vi "PTScanner.dialog edit object.vi"(0 "object ref":refnum<vi>, 2 "Parameters In":T1, 4 "new":bool) -> (14 "object ref out":refnum<vi>, 16 "Parameters Out":T1, 18 "changed":bool)   [LabVIEW 2014, in "PTScanner.lvlib"]
uses:
  PTScanner.lvlib
  _typedefs/scan method parameters/scan method parameters.xctl
  PTScanner.obj parameters.ctl
  _common/PTUtils/PTUtils.lvlib
panel:
  in  "Update button":bool
  in  "different channels":bool caption="diff Channels"
  in  "Channel":i32=-1
  in  "lock address":bool=TRUE caption="locked"
  in  "Range":dbl=1e-15
  in  "dataDescriptor":string caption="Act. Value Service Name"
  in  "cancel":bool
  in  "ok":bool
  in  "Call Mode":enum16{"Simple DIM", "Synchronous"}(ring) caption="Call"
  in  "DIM Services":u16(ring) caption="Services" items=["AG33250A_accessID", "AG33250A_actAmplitude", "AG33250A_actBurstEnabled", "AG33250A_actCycles", "AG33250A_actDCOffset", "AG33250A_actFrequency", "AG33250A_actOutputEnabled", "AG33250A_actPeriod", "AG33250A_actPhase", "AG33250A_actTrigger", "AG33250A_actTriggerDelay", "AG33250A_actWaveform", "AG33250A_birthday", "AG33250A_classID", "AG33250A_condition", "AG33250A_deviceGUI", "AG33250A_deviceID", "AG33250A_deviceState", "AG33250A_eventError", "AG33250A_eventStatus", "AG33250A_evtCounter", "AG33250A_nomAmplitude", "AG33250A_nomBurstEnabled", "AG33250A_nomCycles", "AG33250A_nomDCOffset", "AG33250A_nomFrequency", "AG33250A_nomOutputEnabled", "AG33250A_nomPeriod", "AG33250A_nomPhase", "AG33250A_nomTrigger", "AG33250A_nomTriggerDelay", "AG33250A_nomWaveform", "AG33250A_pdcCounter", "AG33250A_periodicError", "AG33250A_periodicStatus", "AG33250A_systemID", "AG33250A_watchdog"]
  in  "DIM Service":string caption="Act. Value Service Name"
  in  "Method":u16(ring) items=["Ping", "GetDescriptors", "SetPdcInterval", "SetPdcPreset", "SetEvtPreset", "GetEvtStatus", "GetCNames", "GetIList", "Reset", "ReadData", "STOP", "Wait", "WakeupPeriodic", "GetVersionOfLibrary", "Initialize", "Close", "IDQuery", "SetAdvancedGUI", "SetGauss", "UseAM", "ErrorQuery", "SetFrequency", "SetAmplitude", "SetDCOffset", "SetTrigger", "SetBurst", "SetOutputEnabled", "SendTrigger"]
  in  "Object":u16(ring) items=["AG33250A"]
  in  "Step":dbl=1e-15 min=1e-15
  in  "Plus":dbl
  in  "Minus":dbl
  in  "Centroid":dbl
  in  "Method Parameters":T2(xcontrol) caption="Method Input Parameters"
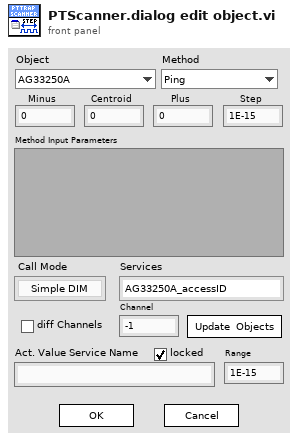
[diagram p1: front panel]
types:
  T1 = typedef "PTScanner.lvlib/PTScanner.obj parameters.ctl" = cluster{"object":string, "DIM address":string, "method":string, "data descriptor":string, "method parameters":cluster{"Name":string, "Descr":string, "Value":string, "Value?":bool}[], "Call Mode":enum16{"Simple DIM", "Synchronous"}, "actValue":dbl, "Centroid":dbl, "Minus Delta":dbl, "Plus Delta":dbl, "increment":dbl, "DIM Status":cluster{"no link":bool, "quality":i32, "Time Stamp":timestamp}, "range":dbl, "DIMChannelIndex":i32}
  T2 = cluster{"Name":string, "Descr":string, "Value":string, "Value?":bool}[]
  T3 = enum8{"Enabled", "Disabled", "Disabled and Grayed Out"}
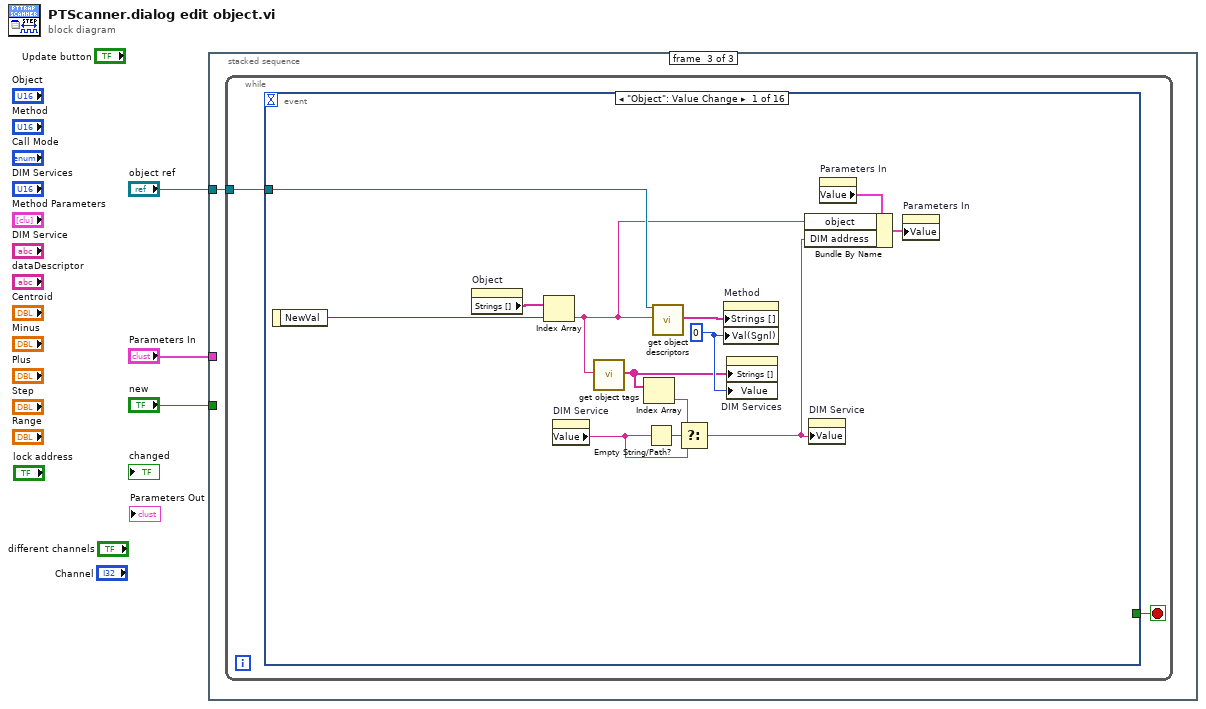
[diagram p0: block diagram]
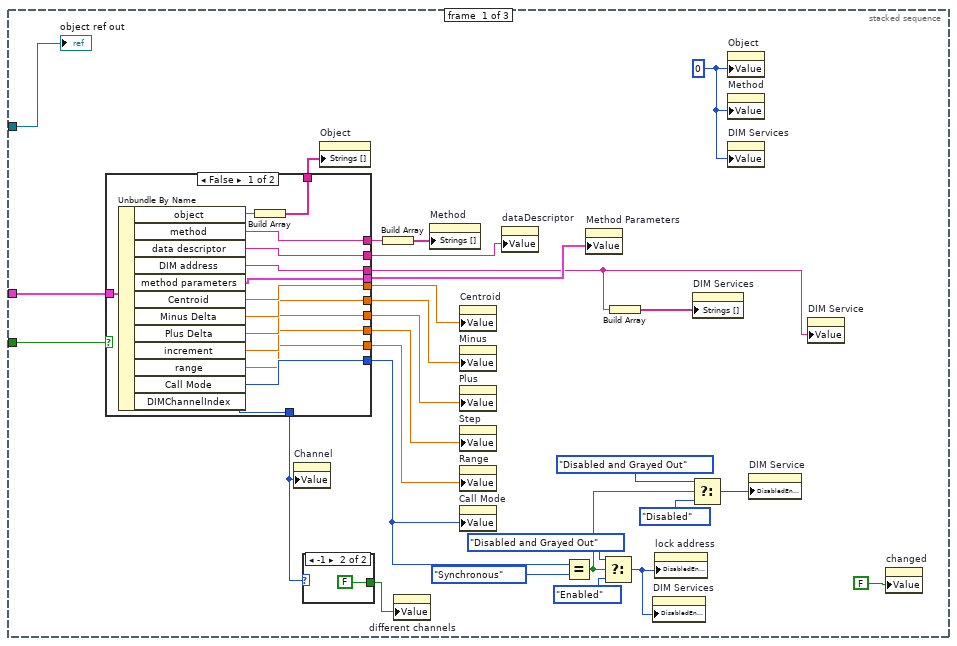
[diagram p2: hidden frame]
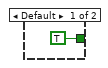
[diagram p3: hidden frame]
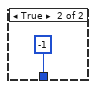
[diagram p4: hidden frame]
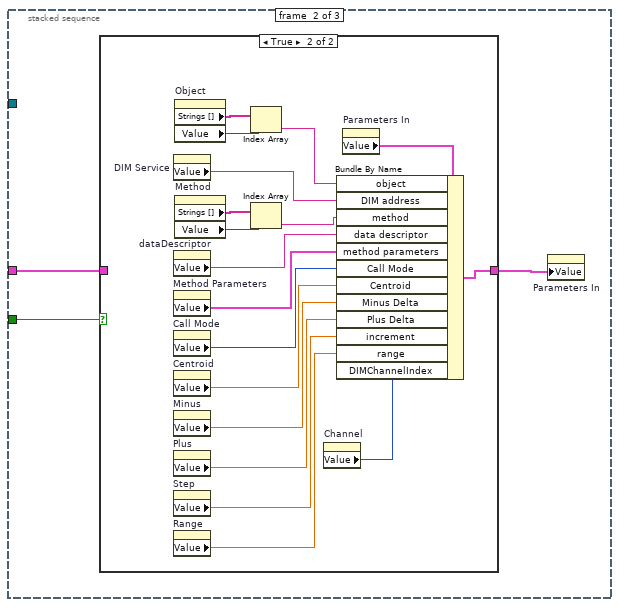
[diagram p5: hidden frame]
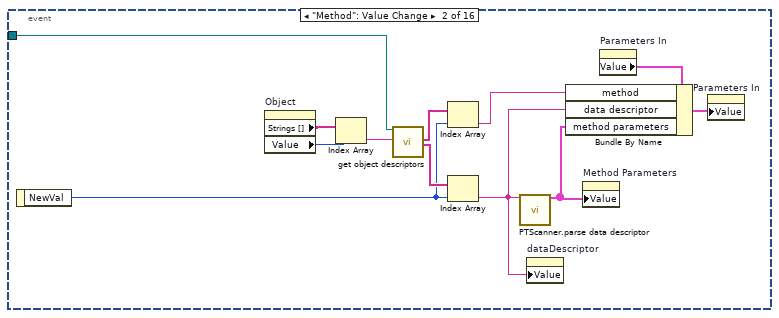
[diagram p7: hidden frame]
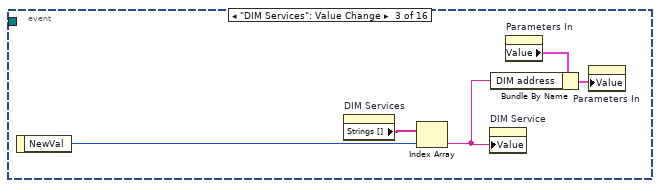
[diagram p8: hidden frame]
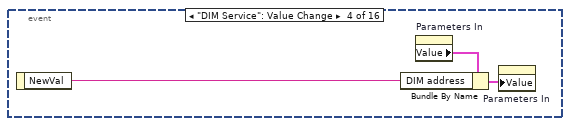
[diagram p9: hidden frame]
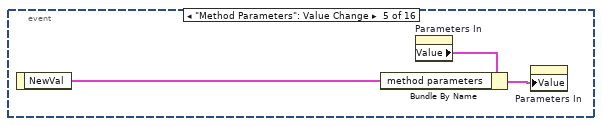
[diagram p10: hidden frame]
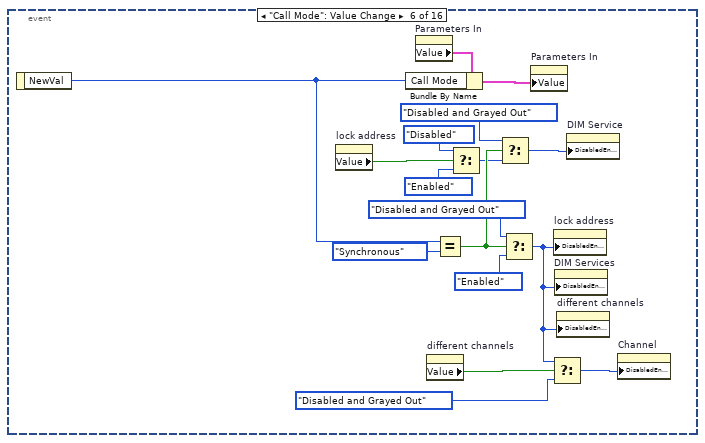
[diagram p11: hidden frame]
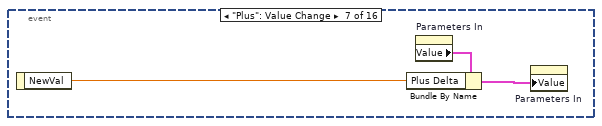
[diagram p12: hidden frame]
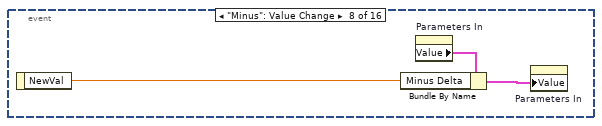
[diagram p13: hidden frame]
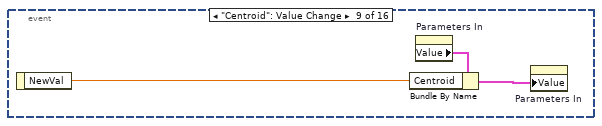
[diagram p14: hidden frame]
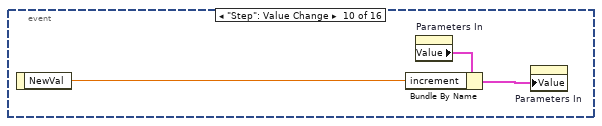
[diagram p15: hidden frame]
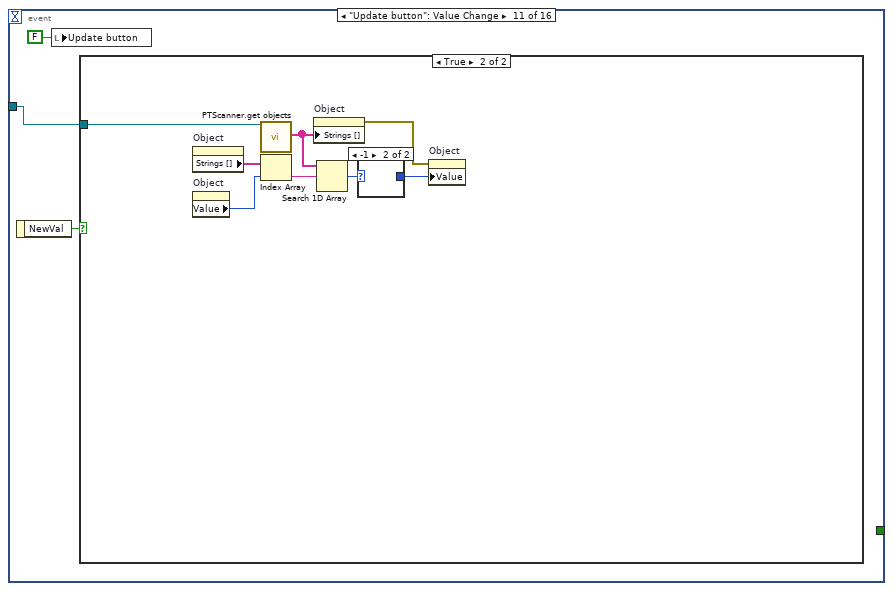
[diagram p16: hidden frame]
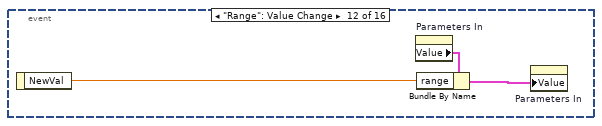
[diagram p19: hidden frame]
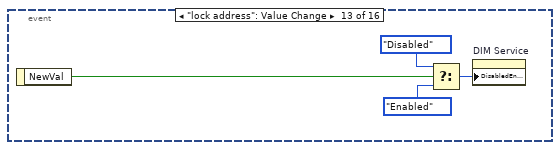
[diagram p20: hidden frame]
diagram:
  n1 = stacked-sequence {
    tunnel: "new" -> [w14 w51 _]
    tunnel: "object ref" -> [w25 _ w71]
    tunnel: "Parameters In" -> [w31 w50 _]
    frame #0 {
      w6 = 0
      n2 = case shown="False" w14 {
        tunnel: w31 -> [w40 _]
        tunnel: [w47 _] -> w10
        tunnel: [w46 _] -> w8
        tunnel: [w45 _] -> w4
        tunnel: [w44 _] -> w30
        tunnel: [w43 _] -> w27
        tunnel: [w42 _] -> w28
        tunnel: [w41 _] -> w29
        tunnel: [w39 _] -> w21
        tunnel: [w38 _] -> w20
        tunnel: [w37 _] -> w7
        tunnel: [w36 -1 ("DIMChannelIndex")] -> w13
        tunnel: [w34 _] -> w11
        frame False {
          n3 = Unbundle By Name(w40) -> ("object"=w35:string, "method"=w47:string, "data descriptor"=w46:string, "DIM address"=w45:string, "method parameters"=w37:T2, "Centroid"=w44:dbl, "Minus Delta"=w43:dbl, "Plus Delta"=w42:dbl, "increment"=w41:dbl, "range"=w38:dbl, "Call Mode"=w39:enum16{"Simple DIM", "Synchronous"}, "DIMChannelIndex"=w36:i32)
          n4 = Build Array(w35) -> (w34:string[])
        }
        frame True {
        }
      }
      n5 = property on="Channel" class="DigNum (strict)"("Value"=w13) -> ()  [unwired: 2 in, 2 out]
      n6 = case shown="-1" w13 {
        tunnel: [TRUE ("changed") FALSE ("changed")] -> w12
        frame Default {
        }
        frame -1 {
        }
      }
      n7 = property on="Object" class="Ring (strict)"("Strings []"=w11) -> ()  [unwired: 2 in, 2 out]
      n8 = Build Array(w10) -> (w9:string[])
      n9 = property on="different channels" class="Bool (strict)"("Value"=w12) -> ()  [unwired: 2 in, 2 out]
      n10 = property on="Method" class="Ring (strict)"("Strings []"=w9) -> ()  [unwired: 2 in, 2 out]
      n11 = property on="Centroid" class="DigNum (strict)"("Value"=w30) -> ()  [unwired: 2 in, 2 out]
      n12 = property on="Minus" class="DigNum (strict)"("Value"=w27) -> ()  [unwired: 2 in, 2 out]
      n13 = property on="Plus" class="DigNum (strict)"("Value"=w28) -> ()  [unwired: 2 in, 2 out]
      n14 = property on="Step" class="DigNum (strict)"("Value"=w29) -> ()  [unwired: 2 in, 2 out]
      n15 = property on="Range" class="DigNum (strict)"("Value"=w20) -> ()  [unwired: 2 in, 2 out]
      n16 = property on="Call Mode" class="Enum (strict)"("Value"=w21) -> ()  [unwired: 2 in, 2 out]
      n17 = property on="dataDescriptor" class="Str"("Value"=w8) -> ()  [unwired: 2 in, 2 out]
      n18 = Equal?(x=w21, y=enum16{"Simple DIM", "Synchronous"}."Synchronous" ("Call Mode")) -> (x = y?=w18:bool)
      n19 = property on="Method Parameters" class="scan method parameters (strict)"("Value"=w7) -> ()  [unwired: 2 in, 2 out]
      n20 = Select(t=T3."Disabled and Grayed Out" ("Disabled"), s=w18, f=T3."Enabled" ("Disabled")) -> (s? t:f=w19:T3)
      n21 = Build Array(w4) -> (w5:string[])
      n22 = property on="DIM Services" class="Ring (strict)"("DisabledEnum"=w19) -> ()  [unwired: 2 in, 2 out]
      n23 = property on="lock address" class="Bool (strict)"("DisabledEnum"=w19) -> ()  [unwired: 2 in, 2 out]
      n24 = Select(t=T3."Disabled and Grayed Out" ("Disabled"), s=w18, f=T3."Disabled" ("Disabled")) -> (s? t:f=w15:T3)
      n25 = property on="DIM Services" class="Ring (strict)"("Strings []"=w5) -> ()  [unwired: 2 in, 2 out]
      n26 = property on="Object" class="Ring (strict)"("Value"=w6) -> ()  [unwired: 2 in, 2 out]
      n27 = property on="Method" class="Ring (strict)"("Value"=w6) -> ()  [unwired: 2 in, 2 out]
      n28 = property on="DIM Services" class="Ring (strict)"("Value"=w6) -> ()  [unwired: 2 in, 2 out]
      n29 = property on="DIM Service" class="Str"("DisabledEnum"=w15) -> ()  [unwired: 2 in, 2 out]
      n30 = property on="DIM Service" class="Str"("Value"=w4) -> ()  [unwired: 2 in, 2 out]
      n31 = property on="changed" class="Bool (strict)"("Value"=FALSE ("changed")) -> ()  [unwired: 2 in, 2 out]
      "object ref out" <- w25
    }
    frame #1 {
      n32 = case shown="True" w51 {
        tunnel: w50 -> [w52 _]
        tunnel: [w52 w65] -> w49
        frame False {
        }
        frame True {
          n33 = property on="DIM Service" class="Str"() -> ("Value"=w63:string)  [unwired: 2 in, 2 out]
          n34 = property on="dataDescriptor" class="Str"() -> ("Value"=w61:string)  [unwired: 2 in, 2 out]
          n35 = property on="Method Parameters" class="scan method parameters (strict)"() -> ("Value"=w60:T2)  [unwired: 2 in, 2 out]
          n36 = property on="Call Mode" class="Enum (strict)"() -> ("Value"=w59:enum16{"Simple DIM", "Synchronous"})  [unwired: 2 in, 2 out]
          n37 = property on="Centroid" class="DigNum (strict)"() -> ("Value"=w58:dbl)  [unwired: 2 in, 2 out]
          n38 = property on="Minus" class="DigNum (strict)"() -> ("Value"=w57:dbl)  [unwired: 2 in, 2 out]
          n39 = property on="Plus" class="DigNum (strict)"() -> ("Value"=w56:dbl)  [unwired: 2 in, 2 out]
          n40 = property on="Step" class="DigNum (strict)"() -> ("Value"=w55:dbl)  [unwired: 2 in, 2 out]
          n41 = property on="Range" class="DigNum (strict)"() -> ("Value"=w54:dbl)  [unwired: 2 in, 2 out]
          n42 = property on="Object" class="Ring (strict)"() -> ("Strings []"=w70:string[], "Value"=w69:u16)  [unwired: 2 in, 2 out]
          n43 = property on="Method" class="Ring (strict)"() -> ("Strings []"=w68:string[], "Value"=w67:u16)  [unwired: 2 in, 2 out]
          n44 = Index Array(array=w70, index=w69) -> (element=w64:string)
          n45 = Index Array(array=w68, index=w67) -> (element=w62:string)
          n46 = property on="Channel" class="DigNum (strict)"() -> ("Value"=w53:i32)  [unwired: 2 in, 2 out]
          n47 = property on="Parameters In" class="Clust (strict)"() -> ("Value"=w66:T1)  [unwired: 2 in, 2 out]
          n48 = Bundle By Name(cluster=w66, "object"=w64, "DIM address"=w63, "method"=w62, "data descriptor"=w61, "method parameters"=w60, "Call Mode"=w59, "Centroid"=w58, "Minus Delta"=w57, "Plus Delta"=w56, "increment"=w55, "range"=w54, "DIMChannelIndex"=w53) -> (w65:T1)
        }
      }
      n49 = property on="Parameters In" class="Clust (strict)"("Value"=w49) -> ()  [unwired: 2 in, 2 out]
    }
    frame #2 {
      n50 = while {
        tunnel: w71 -> [w72]
        stop <- w73 stop-if-true
        n51 = event shown="[0] \"Object\": Value Change" {
          selector: _ -> [_ _ _ _ _ _ _ _ _ _ _ _ _ _ _ _]
          dyn-events: _ -> [_ _ _ _ _ _ _ _ _ _ _ _ _ _ _ _]
          timeout: _ -> [_ _ _ _ _ _ _ _ _ _ _ _ _ _ _ _]
          tunnel: [_ _ _ _ _ _ _ _ _ _ _ _ _ w158 "ok" "cancel"] -> w73
          tunnel: w72 -> [w79 w94 _ _ _ _ _ _ _ _ w139 _ _ _ _ _]
          event "Object": Value Change {
            w81 = u16 0
            n52 = event-data() -> ("NewVal"=w78:u16)  [unwired: 1 in]
            n53 = property on="Object" class="Ring (strict)"() -> ("Strings []"=w83:string[])  [unwired: 2 in, 2 out]
            n54 = Index Array(array=w83, index=w78) -> (element=w75:string)
            n55 = property on="DIM Service" class="Str"() -> ("Value"=w84:string)  [unwired: 2 in, 2 out]
            n56 = call "get object tags.vi"("Object"=w75) -> ("services"=w80:string[])  [unwired: 16 in, 2 out]
            n57 = Index Array(array=w80) -> (element=w85:string)  [unwired: 1 in]
            n58 = Empty String/Path?(string/path=w84) -> (empty?=w86:bool)
            n59 = call "get object descriptors.vi"("i ref in"=w79, "Object"=w75) -> ("selectors"=w82:string[])  [unwired: 14 in, 3 out]
            n60 = Select(t=w85, s=w86, f=w84) -> (s? t:f=w74:string)
            n61 = property on="Method" class="Ring (strict)"("Strings []"=w82, "Val(Sgnl)"=w81) -> ()  [unwired: 2 in, 2 out]
            n62 = property on="DIM Services" class="Ring (strict)"("Strings []"=w80, "Value"=w81) -> ()  [unwired: 2 in, 2 out]
            n63 = property on="DIM Service" class="Str"("Value"=w74) -> ()  [unwired: 2 in, 2 out]
            n64 = property on="Parameters In" class="Clust (strict)"() -> ("Value"=w77:T1)  [unwired: 2 in, 2 out]
            n65 = Bundle By Name(cluster=w77, "object"=w75, "DIM address"=w74) -> (w76:T1)
            n66 = property on="Parameters In" class="Clust (strict)"("Value"=w76) -> ()  [unwired: 2 in, 2 out]
          }
          event "Method": Value Change {
            n67 = event-data() -> ("NewVal"=w91:u16)  [unwired: 1 in]
            n68 = property on="Object" class="Ring (strict)"() -> ("Strings []"=w97:string[], "Value"=w96:u16)  [unwired: 2 in, 2 out]
            n69 = Index Array(array=w97, index=w96) -> (element=w95:string)
            n70 = call "get object descriptors.vi"("i ref in"=w94, "Object"=w95) -> ("selectors"=w92:string[], "Descriptors"=w98:string[])  [unwired: 14 in, 2 out]
            n71 = Index Array(array=w92, index=w91) -> (element=w90:string)
            n72 = Index Array(array=w98, index=w91) -> (element=w87:string)
            n73 = call "PTScanner.parse data descriptor.vi"("dataDescriptor"=w87) -> ("Input Parameters"=w88:T2)  [unwired: 16 in, 2 out]
            n74 = property on="dataDescriptor" class="Str"("Value"=w87) -> ()  [unwired: 2 in, 2 out]
            n75 = property on="Method Parameters" class="scan method parameters (strict)"("Value"=w88) -> ()  [unwired: 2 in, 2 out]
            n76 = property on="Parameters In" class="Clust (strict)"() -> ("Value"=w93:T1)  [unwired: 2 in, 2 out]
            n77 = Bundle By Name(cluster=w93, "method"=w90, "data descriptor"=w87, "method parameters"=w88) -> (w89:T1)
            n78 = property on="Parameters In" class="Clust (strict)"("Value"=w89) -> ()  [unwired: 2 in, 2 out]
          }
          event "DIM Services": Value Change {
            n79 = event-data() -> ("NewVal"=w102:u16)  [unwired: 1 in]
            n80 = property on="DIM Services" class="Ring (strict)"() -> ("Strings []"=w103:string[])  [unwired: 2 in, 2 out]
            n81 = Index Array(array=w103, index=w102) -> (element=w99:string)
            n82 = property on="DIM Service" class="Str"("Value"=w99) -> ()  [unwired: 2 in, 2 out]
            n83 = property on="Parameters In" class="Clust (strict)"() -> ("Value"=w101:T1)  [unwired: 2 in, 2 out]
            n84 = Bundle By Name(cluster=w101, "DIM address"=w99) -> (w100:T1)
            n85 = property on="Parameters In" class="Clust (strict)"("Value"=w100) -> ()  [unwired: 2 in, 2 out]
          }
          event "DIM Service": Value Change {
            n86 = event-data() -> ("NewVal"=w104:string)  [unwired: 1 in]
            n87 = property on="Parameters In" class="Clust (strict)"() -> ("Value"=w106:T1)  [unwired: 2 in, 2 out]
            n88 = Bundle By Name(cluster=w106, "DIM address"=w104) -> (w105:T1)
            n89 = property on="Parameters In" class="Clust (strict)"("Value"=w105) -> ()  [unwired: 2 in, 2 out]
          }
          event "Method Parameters": Value Change {
            n90 = event-data() -> ("NewVal"=w107:T2)  [unwired: 1 in]
            n91 = property on="Parameters In" class="Clust (strict)"() -> ("Value"=w109:T1)  [unwired: 2 in, 2 out]
            n92 = Bundle By Name(cluster=w109, "method parameters"=w107) -> (w108:T1)
            n93 = property on="Parameters In" class="Clust (strict)"("Value"=w108) -> ()  [unwired: 2 in, 2 out]
          }
          event "Call Mode": Value Change {
            n94 = event-data() -> ("NewVal"=w121:enum16{"Simple DIM", "Synchronous"})  [unwired: 1 in]
            n95 = property on="lock address" class="Bool (strict)"() -> ("Value"=w118:bool)  [unwired: 2 in, 2 out]
            n96 = property on="Parameters In" class="Clust (strict)"() -> ("Value"=w126:T1)  [unwired: 2 in, 2 out]
            n97 = Bundle By Name(cluster=w126, "Call Mode"=w121) -> (w125:T1)
            n98 = property on="different channels" class="Bool (strict)"() -> ("Value"=w113:bool)  [unwired: 2 in, 2 out]
            n99 = Equal?(x=w121, y=enum16{"Simple DIM", "Synchronous"}."Synchronous" ("Call Mode")) -> (x = y?=w120:bool)
            n100 = Select(t=T3."Disabled" ("Disabled"), s=w118, f=T3."Enabled" ("Disabled")) -> (s? t:f=w117:T3)
            n101 = Select(t=T3."Disabled and Grayed Out" ("Disabled"), s=w120, f=w117) -> (s? t:f=w114:T3)
            n102 = Select(t=T3."Disabled and Grayed Out" ("Disabled"), s=w120, f=T3."Enabled" ("Disabled")) -> (s? t:f=w111:T3)
            n103 = property on="Parameters In" class="Clust (strict)"("Value"=w125) -> ()  [unwired: 2 in, 2 out]
            n104 = Select(t=w111, s=w113, f=T3."Disabled and Grayed Out" ("Disabled")) -> (s? t:f=w110:T3)
            n105 = property on="lock address" class="Bool (strict)"("DisabledEnum"=w111) -> ()  [unwired: 2 in, 2 out]
            n106 = property on="DIM Services" class="Ring (strict)"("DisabledEnum"=w111) -> ()  [unwired: 2 in, 2 out]
            n107 = property on="different channels" class="Bool (strict)"("DisabledEnum"=w111) -> ()  [unwired: 2 in, 2 out]
            n108 = property on="DIM Service" class="Str"("DisabledEnum"=w114) -> ()  [unwired: 2 in, 2 out]
            n109 = property on="Channel" class="DigNum (strict)"("DisabledEnum"=w110) -> ()  [unwired: 2 in, 2 out]
          }
          event "Plus": Value Change {
            n110 = event-data() -> ("NewVal"=w127:dbl)  [unwired: 1 in]
            n111 = property on="Parameters In" class="Clust (strict)"() -> ("Value"=w129:T1)  [unwired: 2 in, 2 out]
            n112 = Bundle By Name(cluster=w129, "Plus Delta"=w127) -> (w128:T1)
            n113 = property on="Parameters In" class="Clust (strict)"("Value"=w128) -> ()  [unwired: 2 in, 2 out]
          }
          event "Minus": Value Change {
            n114 = event-data() -> ("NewVal"=w130:dbl)  [unwired: 1 in]
            n115 = property on="Parameters In" class="Clust (strict)"() -> ("Value"=w132:T1)  [unwired: 2 in, 2 out]
            n116 = Bundle By Name(cluster=w132, "Minus Delta"=w130) -> (w131:T1)
            n117 = property on="Parameters In" class="Clust (strict)"("Value"=w131) -> ()  [unwired: 2 in, 2 out]
          }
          event "Centroid": Value Change {
            n118 = event-data() -> ("NewVal"=w133:dbl)  [unwired: 1 in]
            n119 = property on="Parameters In" class="Clust (strict)"() -> ("Value"=w135:T1)  [unwired: 2 in, 2 out]
            n120 = Bundle By Name(cluster=w135, "Centroid"=w133) -> (w134:T1)
            n121 = property on="Parameters In" class="Clust (strict)"("Value"=w134) -> ()  [unwired: 2 in, 2 out]
          }
          event "Step": Value Change {
            n122 = event-data() -> ("NewVal"=w136:dbl)  [unwired: 1 in]
            n123 = property on="Parameters In" class="Clust (strict)"() -> ("Value"=w138:T1)  [unwired: 2 in, 2 out]
            n124 = Bundle By Name(cluster=w138, "increment"=w136) -> (w137:T1)
            n125 = property on="Parameters In" class="Clust (strict)"("Value"=w137) -> ()  [unwired: 2 in, 2 out]
          }
          event "Update button": Value Change {
            n126 = event-data() -> ("NewVal"=w140:bool)  [unwired: 1 in]
            n127 = local write "Update button"(FALSE ("Update button")) -> ()
            n128 = case shown="True" w140 {
              tunnel: w139 -> [_ w142]
              frame False {
              }
              frame True {
                n129 = property on="Object" class="Ring (strict)"() -> ("Strings []"=w147:string[])  [unwired: 2 in, 2 out]
                n130 = property on="Object" class="Ring (strict)"() -> ("Value"=w148:u16)  [unwired: 2 in, 2 out]
                n131 = call "PTScanner.get objects.vi"("i ref in"=w142) -> ("objects"=w143:string[])  [unwired: 18 in]
                n132 = Index Array(array=w147, index=w148) -> (element=w149:string)
                n133 = property on="Object" class="Ring (strict)"("Strings []"=w143) -> (error out=w146:errorcluster)  [unwired: 2 in, 1 out]
                n134 = Search 1D Array(1D array=w143, element=w149) -> (index of element=w144:i32)  [unwired: 1 in]
                n135 = case shown="-1" w144 {
                  selector: w144 -> [w150 _]
                  tunnel: [w150 _] -> w145
                  frame 0, Default {
                  }
                  frame -1 {
                  }
                }
                n136 = property on="Object" class="Ring (strict)"(error in=w146, "Value"=w145) -> ()  [unwired: 1 in, 2 out]
              }
            }
          }
          event "Range": Value Change {
            n137 = event-data() -> ("NewVal"=w151:dbl)  [unwired: 1 in]
            n138 = property on="Parameters In" class="Clust (strict)"() -> ("Value"=w153:T1)  [unwired: 2 in, 2 out]
            n139 = Bundle By Name(cluster=w153, "range"=w151) -> (w152:T1)
            n140 = property on="Parameters In" class="Clust (strict)"("Value"=w152) -> ()  [unwired: 2 in, 2 out]
          }
          event "lock address": Value Change {
            n141 = event-data() -> ("NewVal"=w154:bool)  [unwired: 1 in]
            n142 = Select(t=T3."Disabled" ("Disabled"), s=w154, f=T3."Enabled" ("Disabled")) -> (s? t:f=w155:T3)
            n143 = property on="DIM Service" class="Str"("DisabledEnum"=w155) -> ()  [unwired: 2 in, 2 out]
          }
          event Panel Close? {
            w158 = TRUE
            n144 = event-data() -> ()  [unwired: 1 in, 3 out]
            n145 = event-data("Discard?"=w158) -> ()  [unwired: 1 in, 1 out]
          }
          event "ok": Value Change {
            n146 = event-data() -> ()  [unwired: 1 in, 5 out]
            n147 = stacked-sequence {
              frame #0 {
                n148 = property on="Call Mode" class="Enum (strict)"() -> ("Value"=w160:enum16{"Simple DIM", "Synchronous"})  [unwired: 2 in, 2 out]
                n149 = case shown="\"Simple DIM\", Default" w160 {
                  frame "Simple DIM", Default {
                    n150 = property on="Channel" class="DigNum (strict)"() -> ("Value"=w161:i32)  [unwired: 2 in, 2 out]
                    n151 = property on="Parameters In" class="Clust (strict)"() -> ("Value"=w163:T1)  [unwired: 2 in, 2 out]
                    n152 = Bundle By Name(cluster=w163, "DIMChannelIndex"=w161) -> (w162:T1)
                    n153 = property on="Parameters In" class="Clust (strict)"("Value"=w162) -> ()  [unwired: 2 in, 2 out]
                  }
                  frame "Synchronous" {
                    n154 = property on="Parameters In" class="Clust (strict)"() -> ("Value"=w166:T1)  [unwired: 2 in, 2 out]
                    n155 = Bundle By Name(cluster=w166, "DIM address"="Sync", "DIMChannelIndex"=-1) -> (w167:T1)
                    n156 = property on="Parameters In" class="Clust (strict)"("Value"=w167) -> ()  [unwired: 2 in, 2 out]
                  }
                }
              }
              frame #1 {
                n157 = property on="Parameters In" class="Clust (strict)"() -> ("Value"=w169:T1)  [unwired: 2 in, 2 out]
                n158 = property on="Parameters Out" class="Clust (strict)"() -> ("Value"=w170:T1)  [unwired: 2 in, 2 out]
                n159 = Not Equal?(x=w169, y=w170) -> (x != y?=w168:bool)
                n160 = case shown="True" w168 {
                  tunnel: w169 -> [_ w171]
                  frame False {
                  }
                  frame True {
                    n161 = property on="Parameters Out" class="Clust (strict)"("Value"=w171) -> ()  [unwired: 2 in, 2 out]
                  }
                }
                n162 = property on="changed" class="Bool (strict)"("Value"=w168) -> ()  [unwired: 2 in, 2 out]
              }
            }
          }
          event "cancel": Value Change {
            n163 = event-data() -> ()  [unwired: 1 in, 5 out]
          }
        }
      }
    }
  }
